vi "Read port.vi"(8 "error in (no error)":errorcluster, 11 "VISA TCP in":refnum<class "VISA TCP.lvclass">) -> (0 "error out":errorcluster, 2 "port":u16=502, 3 "VISA TCP out":refnum<class "VISA TCP.lvclass">)   [LabVIEW 2021, in "Sockets.lvlib" / "VISA TCP.lvclass"]
uses:
  VISA TCP.lvclass
  VISA TCP.lvclass/VISA TCP.ctl
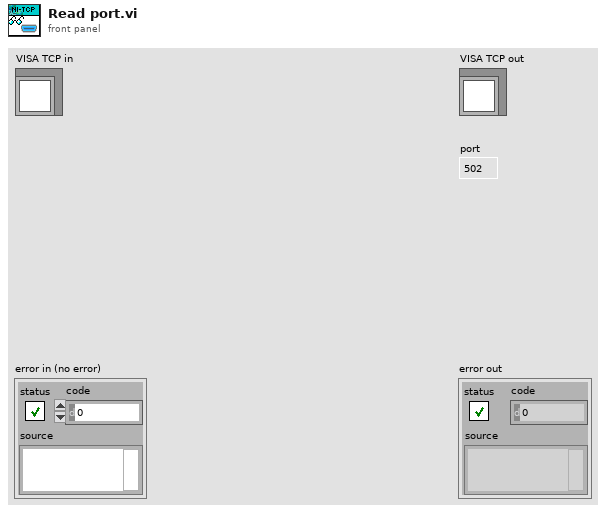
[diagram p1: front panel]
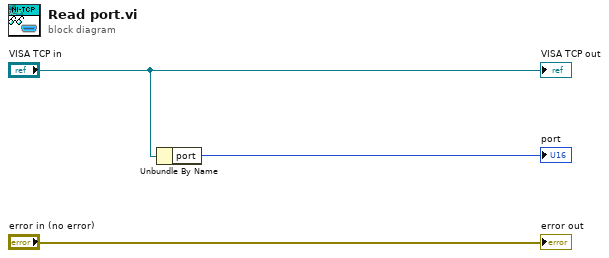
[diagram p0: block diagram]
diagram:
  n1 = Unbundle By Name("VISA TCP in") -> ("port"=→"port":u16)
  "error out" <- "error in (no error)"
  "VISA TCP out" <- "VISA TCP in"
